vi "visa xieru10.23.vi"(4 "Vw":i16, 6 "Vy":i16, 8 "Vx":i16, 9 "工作模式":i32=1, 10 "串口设置（底盘）":T1={"波特率"=115200, "数据位"=8, "校验"=enum."None", "停止位"=10, "流控制"=0} {"流控制" items=["无"=0, "XON/XOFF"=1, "RTS/CTS"=2, "DTR/DSR"=4]; "停止位" items=["1.0"=10, "1.5"=15, "2.0"=20]; "数据位" min=5 max=8 step=1; "波特率" items=["115200"=115200, "460800"=460800, "75"=75, "110"=110, "134"=134, "150"=150, "300"=300, "600"=600, "1200"=1200, "1800"=1800, "2400"=2400, "4800"=4800, "7200"=7200, "9600"=9600, "14400"=14400, "19200"=19200, "28800"=28800, "38400"=38400, "56000"=56000, "57600"=57600, "128000"=128000, "230400"=230400]}, 11 "VISA resource name":refnum<visa-resource-name>="ASRL5::INSTR" caption="VISA资源名称") -> ()   [LabVIEW 2016]
uses:
  <vilib>/Instr/_visa.llb/VISA Configure Serial Port (Instr).vi
panel:
  out "接收数据串/发送串（右1）":string
  out "添加的数组":i32[](array[numeric])
  out "错误输出":errorcluster
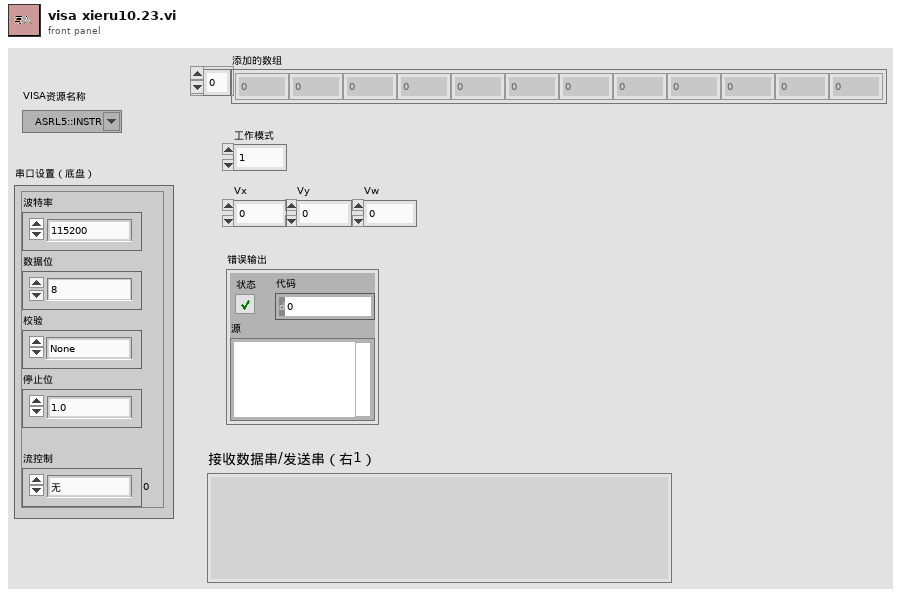
[diagram p1: front panel]
types:
  T1 = cluster{"波特率":u32, "数据位":u16, "校验":enum16{"None", "Odd", "Even", "Mark", "Space"}, "停止位":u16, "流控制":u16}
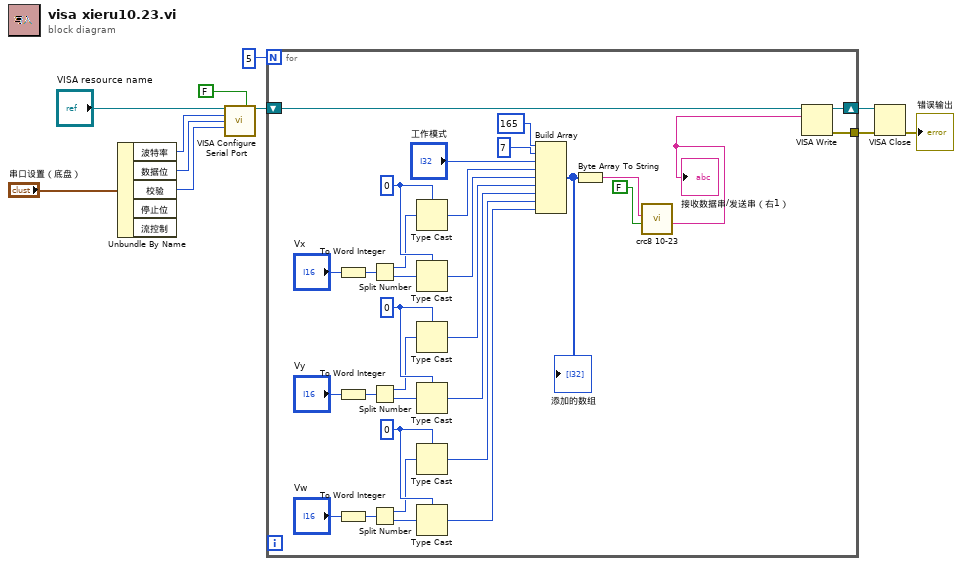
[diagram p0: block diagram]
diagram:
  n1 = Unbundle By Name("串口设置（底盘）") -> ("波特率"=w10:u32, "数据位"=w9:u16, "校验"=w8:enum16{"None", "Odd", "Even", "Mark", "Space"})  [unwired: 2 out]
  n2 = call-poly "VISA Configure Serial Port"("VISA resource name"="VISA resource name", "Enable Termination\nChar (T)"=FALSE ("Enable Termination\nChar (T)"), "baud rate (9600)"=w10, "data bits (8)"=w9, "parity (0:none)"=w8) -> ("VISA resource name out"=w4:refnum<visa-resource-name>)  [unwired: 4 in, 6 out]
  n3 = for {
    N: 5 -> [_]
    tunnel: [w40] -> w2
    shift-right: [w41] -> w3
    shift-left: w4 -> [w42]
    w30 = u8 0
    w34 = u8 0
    w38 = u8 0
    n4 = To Word Integer(number="Vx") -> (16bit integer=w36:i16)
    n5 = To Word Integer(number="Vy") -> (16bit integer=w33:i16)
    n6 = To Word Integer(number="Vw") -> (16bit integer=w29:i16)
    n7 = Split Number(x=w36) -> (hi(x)=w37:u8, lo(x)=w39:u8)
    n8 = Split Number(x=w33) -> (hi(x)=w32:u8, lo(x)=w35:u8)
    n9 = Split Number(x=w29) -> (hi(x)=w28:u8, lo(x)=w31:u8)
    n10 = Type Cast(type=w38, x=w37) -> (*(type *) &x=w20:u8)
    n11 = Type Cast(type=w38, x=w39) -> (*(type *) &x=w19:u8)
    n12 = Type Cast(type=w34, x=w32) -> (*(type *) &x=w18:u8)
    n13 = Type Cast(type=w34, x=w35) -> (*(type *) &x=w17:u8)
    n14 = Type Cast(type=w30, x=w28) -> (*(type *) &x=w16:u8)
    n15 = Type Cast(type=w30, x=w31) -> (*(type *) &x=w15:u8)
    n16 = Build Array(165, 7 ("元素"), "工作模式", w20, w19, w18, w17, w16, w15) -> (w25:i32[])
    "添加的数组" <- w25
    n17 = Byte Array To String(unsigned byte array=w25) -> (string=w14:string)
    n18 = call "crc8 10-23.vi"("功能选择（真读假传）（左2）"=FALSE, "数据输入（左1）"=w14) -> ("接收数据串/发送串（右1）"=w12:string)  [unwired: 9 in]
    "接收数据串/发送串（右1）" <- w12
    n19 = VISA Write(VISA resource name=w42, write buffer=w12) -> (VISA resource name out=w41:refnum<visa-resource-name>, error out=w40:errorcluster)  [unwired: 1 in, 1 out]
  }
  n20 = VISA Close(VISA resource name=w3, error in (no error)=w2) -> (error out=→"错误输出":errorcluster)
